vi "rad_Enable FPGA.vi"(8 "error in (no error)":errorcluster, 10 "device in":refnum<k20>, 11 "session in":refnum<k21>) -> (0 "error out":errorcluster, 2 "device out":refnum<k20>, 3 "session out":refnum<k21>)   [LabVIEW 2020]
uses:
  <vilib>/nisyscfg/Save Changes (Hardware).vi
  <vilib>/nisyscfg/Close (Hardware).vi
  <resource>/objmgr/nisysapi.rc
  <resource>/objmgr/nicontrollersysapi.rc
  <vilib>/nisyscfg/nisyscfg.lvlib
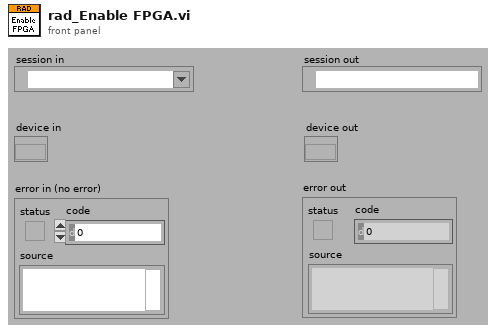
[diagram p1: front panel]
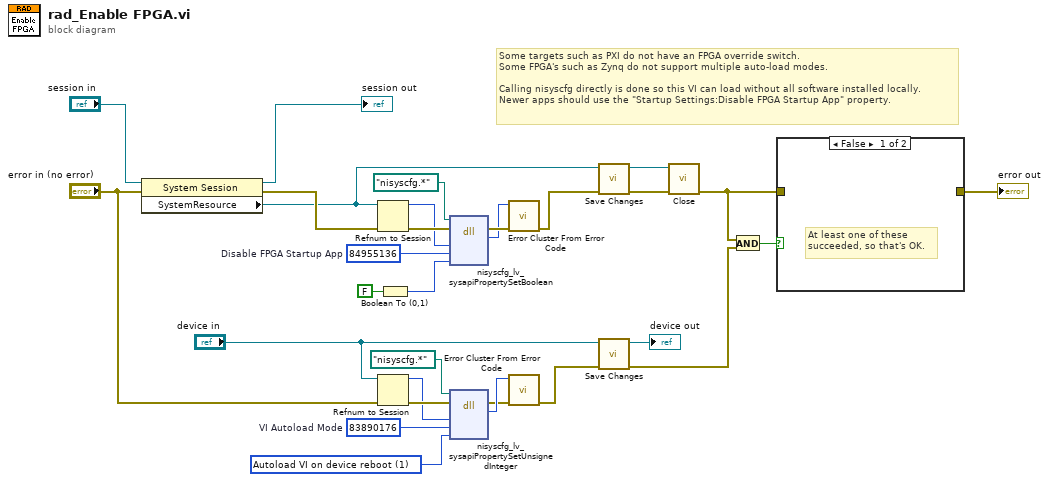
[diagram p0: block diagram]
diagram:
  w12 = u32 83890176  # VI Autoload Mode
  w13 = u32 84955136  # Disable FPGA Startup App
  w11 = u32 1 items=["Do not autoload VI", "Autoload VI on device reboot", "Autoload VI on device powerup"] ("RIO:Flash Access:VI Autoload Mode")
  # "Some targets such as PXI do not have an FPGA override switch.\nSome FPGA's such as Zynq do not support multiple auto-load modes.\n\nCalling nisyscfg directly is done so this VI can load without all software installed locally.\nNewer apps should use the \"Startup Settings:Disable FPGA Startup App\" property."
  n1 = property class="System Session"(reference="session in", error in="error in (no error)") -> (reference out=→"session out":refnum<k21>, error out=w7:errorcluster, "SystemResource"=w1:refnum<k20>)
  n2 = Refnum to Session(4:w7, 7:w1) -> (0:w21:errorcluster, 3:w3:u64)
  n3 = Refnum to Session(4:"error in (no error)", 7:"device in") -> (0:w14:errorcluster, 3:w4:u64)
  n4 = Boolean To (0,1)(Boolean=FALSE ("Startup Settings:Disable RT Startup App")) -> (0, 1=w9:i16)
  n5 = dll-call lib="nisyscfg.dll" fn="nisyscfg_lv_sysapiPropertySetBoolean"(path in=path "nisyscfg.*", error in=w21, "resource"=w3, "attribute"=w13, "value"=w9) -> (error out=w20:errorcluster, "status"=w18:i32)  [unwired: 4 in, 1 out]
  n6 = dll-call lib="nisyscfg.dll" fn="nisyscfg_lv_sysapiPropertySetUnsignedInteger"(path in=path "nisyscfg.*", error in=w14, "resource"=w4, "attribute"=w12, "value"=w11) -> (error out=w15:errorcluster, "status"=w17:i32)  [unwired: 4 in, 1 out]
  n7 = call <vilib>:"Error Cluster From Error Code.vi"("error in (no error)"=w20, "error code (0)"=w18) -> ("error out"=w2:errorcluster)  [unwired: 2 in, 5 out]
  n8 = call <vilib>:"Error Cluster From Error Code.vi"("error in (no error)"=w15, "error code (0)"=w17) -> ("error out"=w6:errorcluster)  [unwired: 1 in, 6 out]
  n9 = call-poly <vilib>:"Save Changes.vi"("error in (no error)"=w2, "Resource in"=w1) -> ("error out"=w27:errorcluster, "Resource out"=w28:refnum<k20>)  [unwired: 6 in, 2 out]
  n10 = call-poly <vilib>:"Save Changes.vi"("error in (no error)"=w6, "Resource in"="device in") -> ("error out"=w23:errorcluster, "Resource out"=→"device out":refnum<k20>)  [unwired: 6 in, 2 out]
  n11 = call-poly <vilib>:"Close.vi"("error in (no error)"=w27, "Resource in"=w28) -> ("error out"=w24:errorcluster)  [unwired: 9 in]
  n12 = And(x=w24, y=w23) -> (x .and. y?=w22:bool)
  n13 = case shown="False" w22 {
    tunnel: w24 -> [_ w31]
    tunnel: [_ w31] -> w25
    frame False {
      # "At least one of these\nsucceeded, so that's OK."
    }
    frame True {
      # "Both failed, so just\nreturn the first error."
    }
  }
  "error out" <- w25
